vi "Initialize Producer.vi"(8 "error in (no error)":errorcluster, 11 "Engine Data in":T1) -> (0 "error out":errorcluster, 3 "Engine Data out":T1)   [LabVIEW 2019, in "Routing and Faulting Engine.lvlib"]
uses:
  Routing and Faulting Engine.lvlib
  Engine Data.ctl
  Includes/CDMessaging.lvlibp/Producer/Abstract Producer/Abstract Producer.lvclass
  Shared/Compiled.Settings.ctl
  Shared/Communication Configuration.ctl
  Shared/Routing and Faulting Configuration.ctl
  Shared/Routing Channel Configuration.ctl
  Shared/Value-Connections Map.ctl
  Shared/Alias Mapping.ctl
  Shared/Alias Endpoint.ctl
  Shared/Compiled Connection.ctl
  Shared/FIFO Indices.ctl
  Device Inputs.ctl
  Device Outputs.ctl
  Includes/CDMessaging.lvlibp/Parameters/Abstract Init Parameters/Abstract Init Parameters.lvclass
  Includes/CDMessaging.lvlibp/Message Queue/Message Queue/Message Queue.lvclass
  C:/Dev/GitHub/niveristand-routing-and-faulting-custom-device/Includes/CDMessaging.lvlibp/Message Queue/Abstract Message Queue/Abstract Message Queue.lvclass
  Shared/Routing and Faulting Shared.lvlib
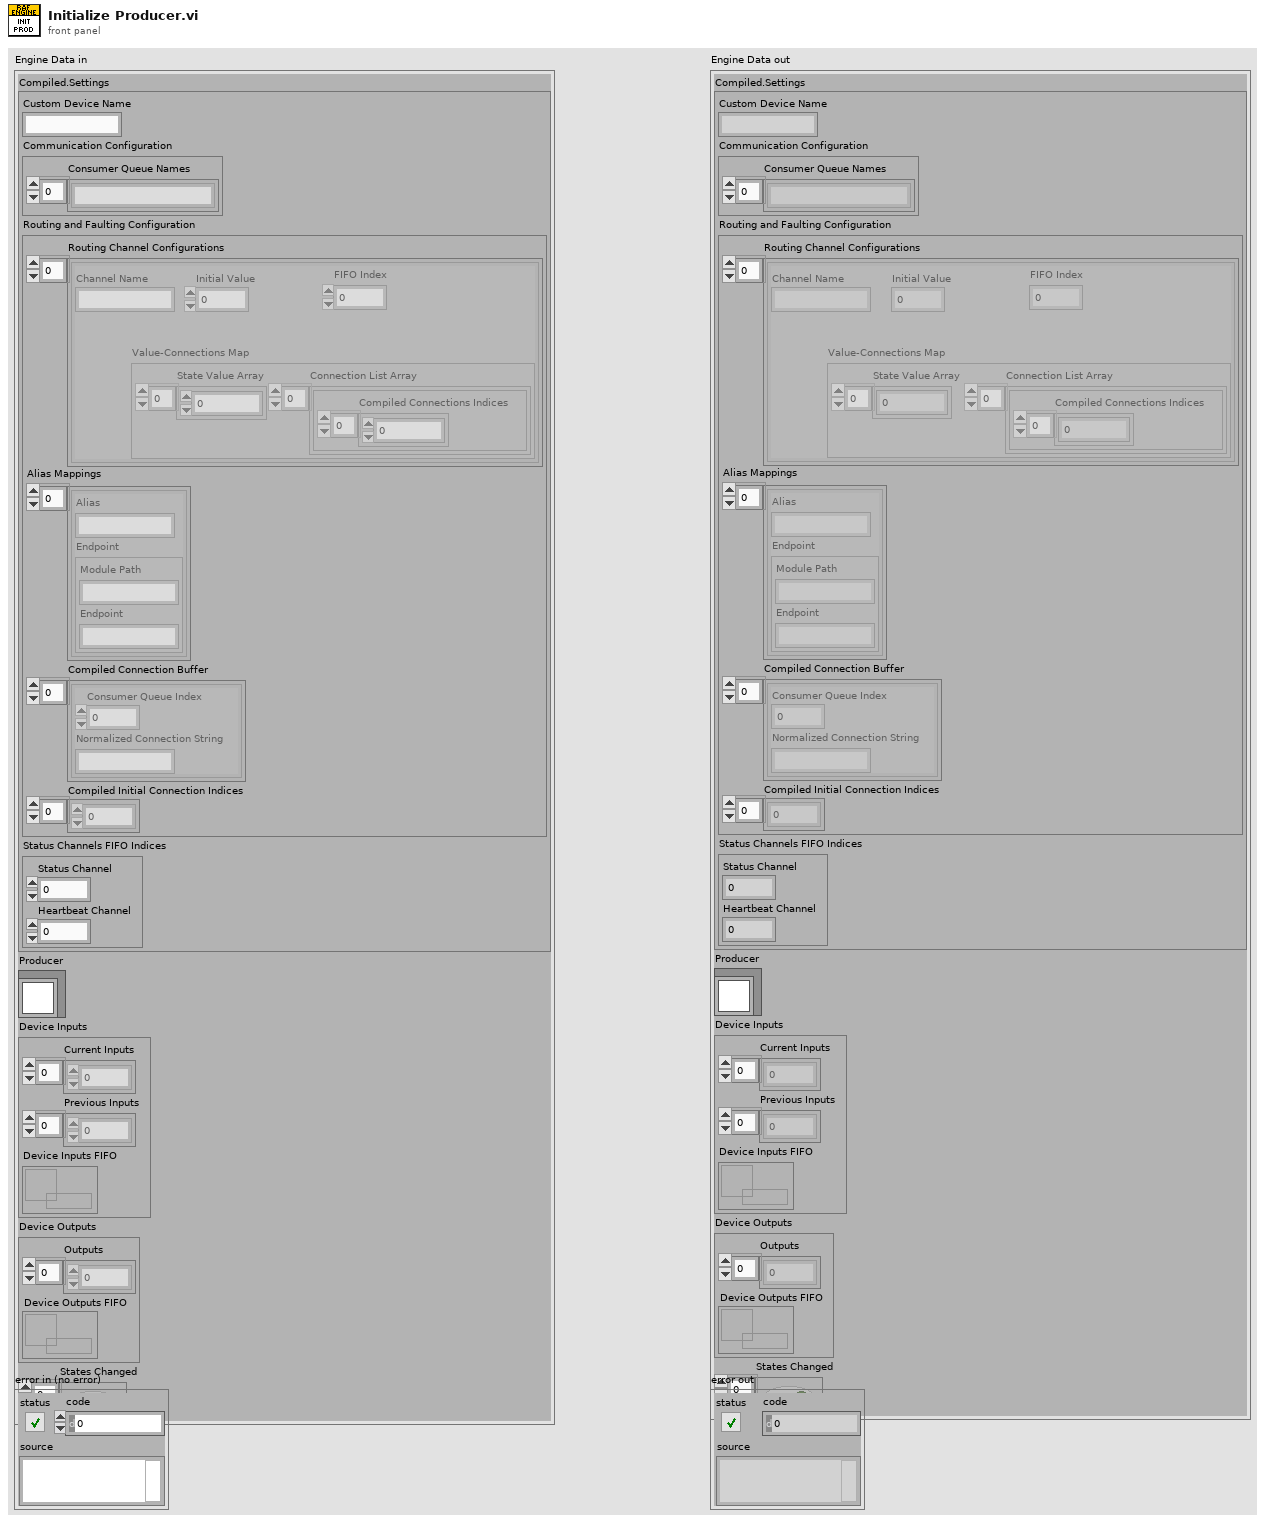
[diagram p1: front panel]
types:
  T1 = typedef "Routing and Faulting Engine.lvlib/Engine Data.ctl" = cluster{"Compiled.Settings":T2, "Producer":refnum<class "Abstract Producer.lvclass">, "Device Inputs":T11, "Device Outputs":T12, "States Changed":bool[]}
  T2 = typedef "Routing and Faulting Shared.lvlib/Compiled.Settings.ctl" = cluster{"Custom Device Name":string, "Communication Configuration":T3, "Routing and Faulting Configuration":T4, "Status Channels FIFO Indices":T10}
  T3 = typedef "Routing and Faulting Shared.lvlib/Communication Configuration.ctl" = cluster{"Consumer Queue Names":string[]}
  T4 = typedef "Routing and Faulting Shared.lvlib/Routing and Faulting Configuration.ctl" = cluster{"Routing Channel Configurations":T5[], "Alias Mappings":T7[], "Compiled Connection Buffer":T9[], "Compiled Initial Connection Indices":i32[]}
  T5 = typedef "Routing and Faulting Shared.lvlib/Routing Channel Configuration.ctl" = cluster{"Channel Name":string, "Initial Value":dbl, "FIFO Index":i32, "Value-Connections Map":T6}
  T6 = typedef "Routing and Faulting Shared.lvlib/Value-Connections Map.ctl" = cluster{"State Value Array":i32[], "Connection List Array":cluster{"Compiled Connections Indices":i32[]}[]}
  T7 = typedef "Routing and Faulting Shared.lvlib/Alias Mapping.ctl" = cluster{"Alias":string, "Endpoint":T8}
  T8 = typedef "Routing and Faulting Shared.lvlib/Alias Endpoint.ctl" = cluster{"Module Path":string, "Endpoint":string}
  T9 = typedef "Routing and Faulting Shared.lvlib/Compiled Connection.ctl" = cluster{"Consumer Queue Index":i32, "Normalized Connection String":string}
  T10 = typedef "Routing and Faulting Shared.lvlib/FIFO Indices.ctl" = cluster{"Status Channel":i32, "Heartbeat Channel":i32}
  T11 = typedef "Routing and Faulting Engine.lvlib/Device Inputs.ctl" = cluster{"Current Inputs":dbl[], "Previous Inputs":dbl[], "Device Inputs FIFO":refnum<k33>}
  T12 = typedef "Routing and Faulting Engine.lvlib/Device Outputs.ctl" = cluster{"Outputs":dbl[], "Device Outputs FIFO":refnum<k33>}
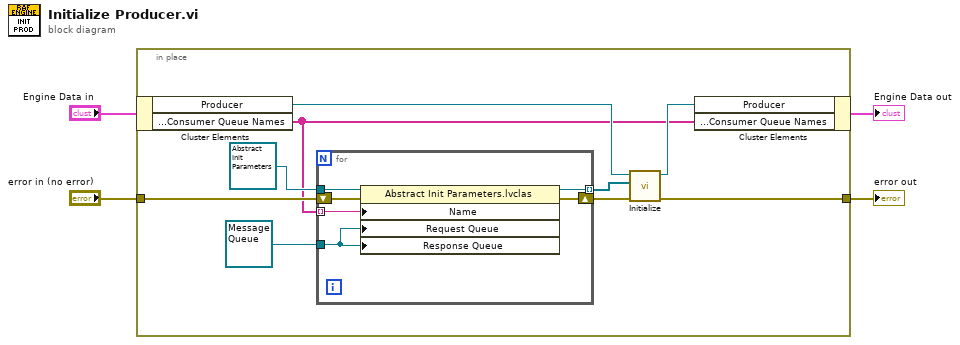
[diagram p0: block diagram]
diagram:
  n1 = in-place {
    in-place-border: "error in (no error)" -> [w8]
    in-place-border: [w5] -> w2
    n2 = in-place-cluster #1("Engine Data in") -> ("Producer"=w11:refnum<class "Abstract Producer.lvclass">, "Compiled.Settings.Communication Configuration.Consumer Queue Names"=w6:string[])
    n3 = for {
      tunnel: refnum<class "Abstract Init Parameters.lvclass"> refnum ("CDMessaging.lvlibp:Abstract Init Parameters.lvclass") -> [w19]
      tunnel: refnum<class "Message Queue.lvclass"> refnum ("CDMessaging.lvlibp:Message Queue.lvclass") -> [w18]
      tunnel: w6 -> [w17] mode=indexing
      tunnel: [w16] -> w10 mode=indexing
      shift-right: [w14] -> w7
      shift-left: w8 -> [w15]
      n4 = property class="Abstract Init Parameters.lvclas"(reference=w19, error in=w15, "Name"=w17, "Request Queue"=w18, "Response Queue"=w18) -> (reference out=w16:refnum<class "Abstract Init Parameters.lvclass">, error out=w14:errorcluster)
    }
    n5 = call "Initialize.vi"("error in (no error)"=w7, "Parameters in"=w10, "Abstract Producer in"=w11) -> ("error out"=w5:errorcluster, "Abstract Producer out"=w9:refnum<class "Abstract Producer.lvclass">)  [unwired: 7 in]
    n6 = in-place-cluster #1("Producer"=w9, "Compiled.Settings.Communication Configuration.Consumer Queue Names"=w6) -> (→"Engine Data out":T1)
  }
  "error out" <- w2
